vi "Choose error bar type.vi"(2 "Error_bars":T1, 3 "Error Bar Type":T2) -> (0 "Lower":string[](array[string]), 1 "Upper":string[](array[string]))   [LabVIEW 2016]
uses:
  Error bar Type.ctl
  Error_bars.ctl
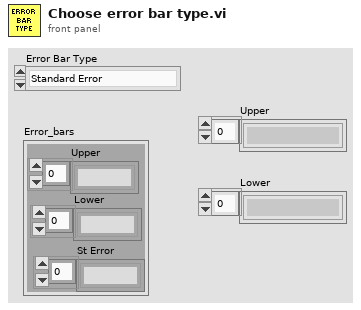
[diagram p1: front panel]
types:
  T1 = typedef "Error_bars.ctl" = cluster{"Upper":string[], "Lower":string[], "St Error":string[]}
  T2 = typedef "Error bar Type.ctl" = enum16{"Standard Error", "Separate upper and lower"}
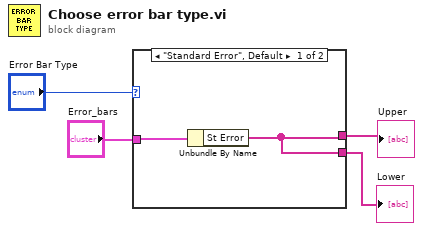
[diagram p0: block diagram]
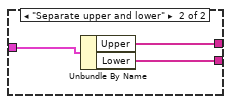
[diagram p2: hidden frame]
diagram:
  n1 = case shown="\"Standard Error\", Default" "Error Bar Type" {
    tunnel: "Error_bars" -> [w6 w9]
    tunnel: [w5 w8] -> w2
    tunnel: [w5 w7] -> w1
    frame "Standard Error", Default {
      n2 = Unbundle By Name(w6) -> ("St Error"=w5:string[])
    }
    frame "Separate upper and lower" {
      n3 = Unbundle By Name(w9) -> ("Upper"=w8:string[], "Lower"=w7:string[])
    }
  }
  "Upper" <- w2
  "Lower" <- w1
